vi "git_export.vi"   [LabVIEW 2023]
uses:
  <vilib>/Hampel Software Engineering/Git API/Source/Git API/GIT-api.lvclass
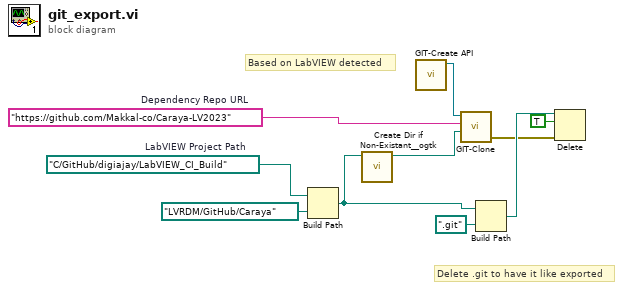
[diagram p0: block diagram]
diagram:
  w9 = path "C:/GitHub/digiajay/LabVIEW_CI_Build"  # LabVIEW Project Path
  w10 = "https://github.com/Makkal-co/Caraya-LV2023"  # Dependency Repo URL
  # "Delete .git to have it like exported"
  # "Based on LabVIEW detected"
  n1 = Build Path(base path=w9, name or relative path=path "LVRDM/GitHub/Caraya") -> (appended path=w5:path)
  n2 = call <userlib>:"Create Dir if Non-Existant__ogtk.vi"("Directory Path"=w5) -> ("dup Directory Path"=w6:path)  [unwired: 8 in, 2 out]
  n3 = call <vilib>:"GIT-Create API.vi"() -> ("git-api out"=w7:refnum<class "GIT-api.lvclass">)  [unwired: 10 in, 1 out]
  n4 = call <vilib>:"GIT-Clone.vi"("Local Path"=w6, "Repository URL"=w10, "git-api in"=w7) -> ("error out"=w2:errorcluster)  [unwired: 6 in, 2 out]
  n5 = Build Path(base path=w5, name or relative path=path ".git") -> (appended path=w3:path)
  n6 = Delete(path (use dialog)=w3, entire hierarchy (F)=TRUE, error in=w2) -> ()  [unwired: 2 in, 3 out]
